vi "FS Sketch Polyline.vi"(8 "Sketch #":i32=1, 9 "Polyline Points":dbl[][](array[numeric]), 10 "Sketch Plane":T1, 11 "Feature In":string="FeatureScript 1247;\nimport(path : \"onshape/std/geometry.fs\", version : \"1247.0\");\n\nannotation { \"Feature Type Name\" : \"LabVIEW Feature\" }\nexport const myFeature = defineFeature(function(context is Context, id is Id, definition is map)\n    precondition\n    {\n        // Define the parameters of the feature type\n    }\n    {\n        // Define the function's action\n    });") -> (3 "Feature Out":string="FeatureScript 1247;\nimport(path : \"onshape/std/geometry.fs\", version : \"1247.0\");\n\nannotation { \"Feature Type Name\" : \"LVFeat1\" }\nexport const myFeature = defineFeature(function(context is Context, id is Id, definition is map)\n    precondition\n    {\n        // Define the parameters of the feature type\n    }\n    {\n        // Define the function's action\n\nvar sketch1 = newSketch(context, id + \"sketch1\", {\n                \"sketchPlane\" : qCreatedBy(makeId(\"Top\"), EntityType.FACE)\n        });\n        // Create sketch entities here\n        skRectangle(sketch1, \"rectangle1\", {\n                \"firstCorner\" : vector(0, 0) * inch,\n                \"secondCorner\" : vector(3, 4) * inch\n        });\n        \n        skSolve(sketch1);\n    });")   [LabVIEW 2019]
uses:
  Users/matt/Documents/LabVIEW/Sketch Plane.ctl
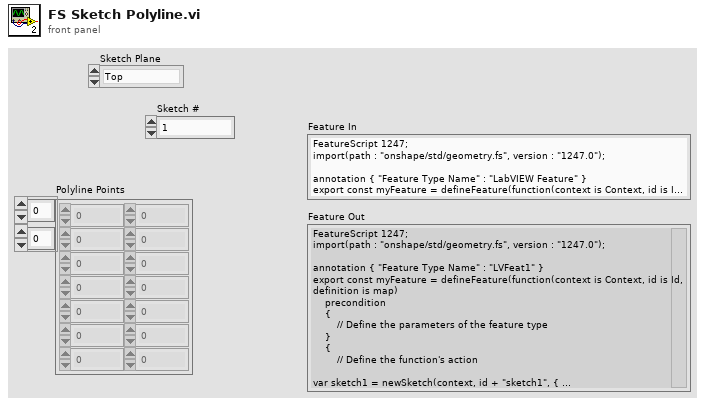
[diagram p1: front panel]
types:
  T1 = typedef "Sketch Plane.ctl" = enum16{"Top", "Front", "Right", "plane1", "plane2", "plane3"}
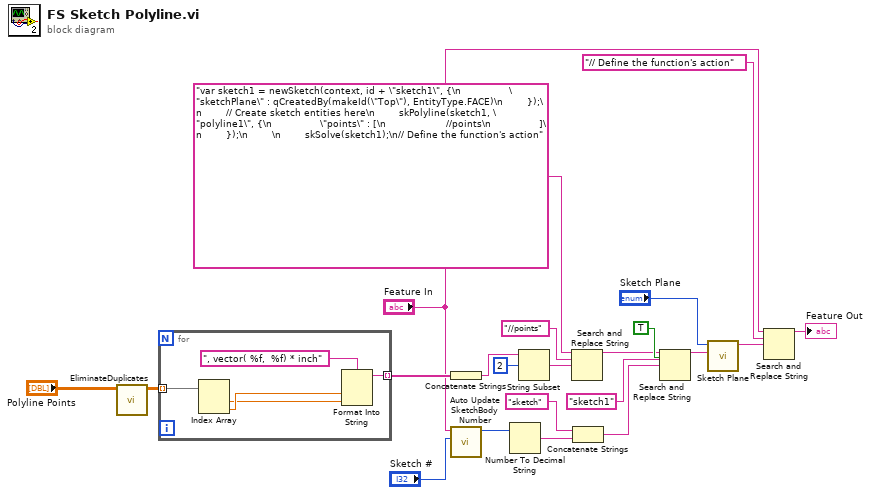
[diagram p0: block diagram]
diagram:
  n1 = call "EliminateDuplicates.vi"("Polyline Points in"="Polyline Points") -> ("Polyline Points out"=w1:dbl[][])  [unwired: 10 in]
  n2 = for {
    tunnel: w1 -> [w27] mode=indexing
    tunnel: [w25] -> w12 mode=indexing
    n3 = Index Array(array=w27) -> (element #1=w23:dbl, element #2=w24:dbl)  [unwired: 2 in]
    n4 = Format Into String(format string=", vector( %f,  %f) * inch" ("string"), w24, w23) -> (resulting string=w25:string)  [unwired: 2 in, 1 out]
  }
  n5 = Concatenate Strings(w12) -> (w11:string)
  n6 = call <userlib>:"Auto Update SketchBody Number.vi"("Sketch # in"="Sketch #", "Feature In"="Feature In") -> ("Sketch # out"=w4:i32)  [unwired: 8 in, 1 out]
  n7 = Number To Decimal String(number=w4) -> (decimal integer string=w14:string)  [unwired: 1 in]
  n8 = String Subset(string=w11, offset (0)=2) -> (substring=w9:string)  [unwired: 1 in]
  n9 = Search and Replace String(input string="var sketch1 = newSketch(context, id + \"sketch1\", {\n                \"sketchPlane\" : qCreatedBy(makeId(\"Top\"), EntityType.FACE)\n        });\n        // Create sketch entities here\n        skPolyline(sketch1, \"polyline1\", {\n                \"points\" : [\n                    //points\n                ]\n        });\n        \n        skSolve(sketch1);\n// Define the function's action" ("string"), search string="//points" ("regular expression"), replace string=w9) -> (result string=w13:string)  [unwired: 5 in, 3 out]
  n10 = Concatenate Strings("sketch" ("regular expression"), w14) -> (w15:string)
  n11 = Search and Replace String(replace all?=TRUE ("replace all? (F)"), input string=w13, search string="sketch1" ("regular expression"), replace string=w15) -> (result string=w8:string)  [unwired: 4 in, 3 out]
  n12 = call <userlib>:"Sketch Plane.vi"("result string in"=w8, "Sketch Plane"="Sketch Plane") -> ("result string out"=w6:string)  [unwired: 9 in]
  n13 = Search and Replace String(input string="Feature In", search string="// Define the function's action", replace string=w6) -> (result string=→"Feature Out":string)  [unwired: 5 in, 3 out]
